vi "Get Resistance Waveform.vi"(10 "Channel config":T2={"Voltage channel index"=1, "Current channel index"=2}, 11 "array":waveform(dbl)[](array[waveform])) -> (2 "Resistance waveform out":waveform(dbl), 4 "Channel names":T1)   [LabVIEW 2019]
doc: "This example demonstrates how to acquire a continuous amount of data (Waveform) using the DAQ device's internal clock. It also shows how to synchronize two devices for different device families (E Series, S Series, M Series, X Series, DSA, and SC Express), to simultaneously acquire the data.\n\nFor instructions on how to connect your signals to the DAQ device, refer to your device documentation."
panel:
  # "Get Resistance Waveform"
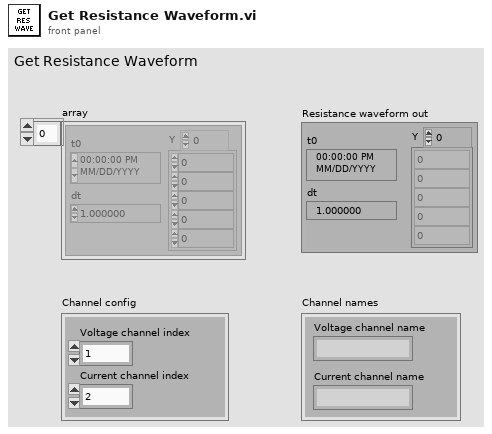
[diagram p1: front panel]
types:
  T1 = cluster{"Voltage channel name":string, "Current channel name":string}
  T2 = cluster{"Voltage channel index":i32, "Current channel index":i32}
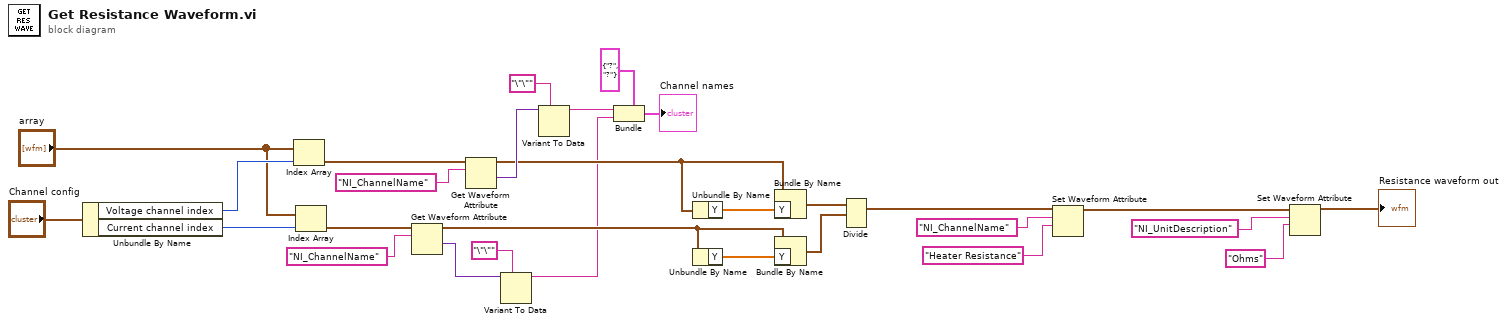
[diagram p0: block diagram]
diagram:
  n1 = Unbundle By Name("Channel config") -> ("Voltage channel index"=w25:i32, "Current channel index"=w21:i32)
  n2 = Index Array(array="array", index=w25) -> (element=w29:waveform(dbl))
  n3 = Index Array(array="array", index=w21) -> (element=w16:waveform(dbl))
  n4 = Get Waveform Attribute(6:"NI_ChannelName" ("name"), 7:w16) -> (1:w17:variant, 3:w14:waveform(dbl))  [unwired: 2 in, 2 out]
  n5 = Get Waveform Attribute(6:"NI_ChannelName" ("name"), 7:w29) -> (1:w24:variant, 3:w23:waveform(dbl))  [unwired: 2 in, 2 out]
  n6 = Variant To Data(type="\"\"" ("name"), Variant=w17) -> (data=w4:string)  [unwired: 1 in, 1 out]
  n7 = Variant To Data(type="\"\"" ("name"), Variant=w24) -> (data=w5:string)  [unwired: 1 in, 1 out]
  n8 = Bundle(cluster=cluster{"name":string, "name":string} {"name"="?", "name"="?"}, "name"=w5, "name"=w4) -> (→"Channel names":cluster{"name":string, "name":string})
  n9 = Unbundle By Name(w23) -> ("Y"=w22:dbl[])
  n10 = Unbundle By Name(w14) -> ("Y"=w15:dbl[])
  n11 = Bundle By Name(cluster=w23, "Y"=w22) -> (w7:waveform(dbl))
  n12 = Bundle By Name(cluster=w14, "Y"=w15) -> (w1:waveform(dbl))
  n13 = Divide(1:w1, 2:w7) -> (0:w6:waveform(dbl))  [unwired: 1 in, 1 out]
  n14 = Set Waveform Attribute(5:"Heater Resistance" ("name"), 6:"NI_ChannelName" ("name"), 7:w6) -> (3:w11:waveform(dbl))  [unwired: 1 in, 2 out]
  n15 = Set Waveform Attribute(5:"Ohms" ("name"), 6:"NI_UnitDescription" ("name"), 7:w11) -> (3:→"Resistance waveform out":waveform(dbl))  [unwired: 1 in, 2 out]
